vi "Newport PM-USB Dual CH 2936R.vi"(0 "Device State Control":T2, 1 "2936R Ref In":refnum<k24>, 5 "USB Address":i32=1, 7 "Remote Msg On":bool, 9 "PowerMeter 2936R Settings":T1={"Wavelength nm"=266, "Range Select"=0, "Mode"=0, "Unit Select"=2, "Auto Select"=1, "Analog Filter"=0, "Digital Filter\n(int. 0 to 10000)"=0, "Filter"=0} {"Filter" items=["No filtering", "Analog filter", "Digital filter", "Analog and Digital filter"]; "Digital Filter\n(int. 0 to 10000)" min=0 max=10000; "Analog Filter" items=["None", "250 kHz", "12.5 kHz", "1 kHz", "5 kHz"]; "Auto Select" items=["Manual Range", "Auto Range"]; "Unit Select" items=["Amps", "Volts", "Watts", "Watts/cm2", "Joules", "Joules/cm2", "dBm"]; "Mode" items=["CW Cont.", "DC Single", "Integrate", "Peak-to-Peak Cont.", "Peak-to-Peak Single", "Pulse Continuous", "Pulse Single", "RMS"]; "Range Select" items=["Range 0", "Range 1", "Range 2", "Range 3", "Range 4", "Range 5", "Range 6", "Range 7"]; "Wavelength nm" min=0}, 11 "2936R error in":errorcluster, 12 "Msg Ctl Refnum":refnum<vi>) -> (3 "2936R Ref Out":refnum<k24>, 4 "CH1, W":dbl, 6 "Ch2, W":dbl, 8 "Open USB IDs":string, 10 "Msg":string="\n\r" caption="Status", 13 "Error":bool, 14 "2936R Open?":bool, 15 "2936R error out":errorcluster)   [LabVIEW 2017]
uses:
  C:/Program Files (x86)/Newport/Newport USB Driver/Bin/UsbDllWrap.dll
  Program Files (x86)/Newport/Newport USB Driver/Bin/UsbDllWrap.dll
  Device State Control.ctl
panel:
  in  "Enable Error Reporting":bool=TRUE
  # "Model 1931-C|1936-C = Single Channel\nModel 2936-R = Dual Channel"
  # "Dual channel 2936R settings and power reading command"
  # "Ref out after init"
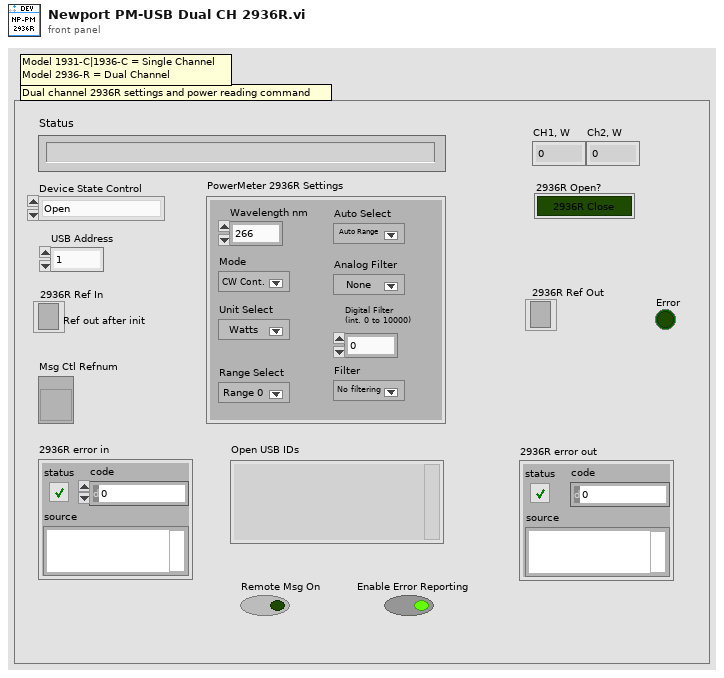
[diagram p1: front panel]
types:
  T1 = cluster{"Wavelength nm":i32, "Range Select":i32, "Mode":i32, "Unit Select":i32, "Auto Select":i32, "Analog Filter":i32, "Digital Filter\n(int. 0 to 10000)":i32, "Filter":i32}
  T2 = typedef "Device State Control.ctl" = enum16{"Open", "Close", "Clear", "Set", "Reset", "Read", "Write", "Call"}
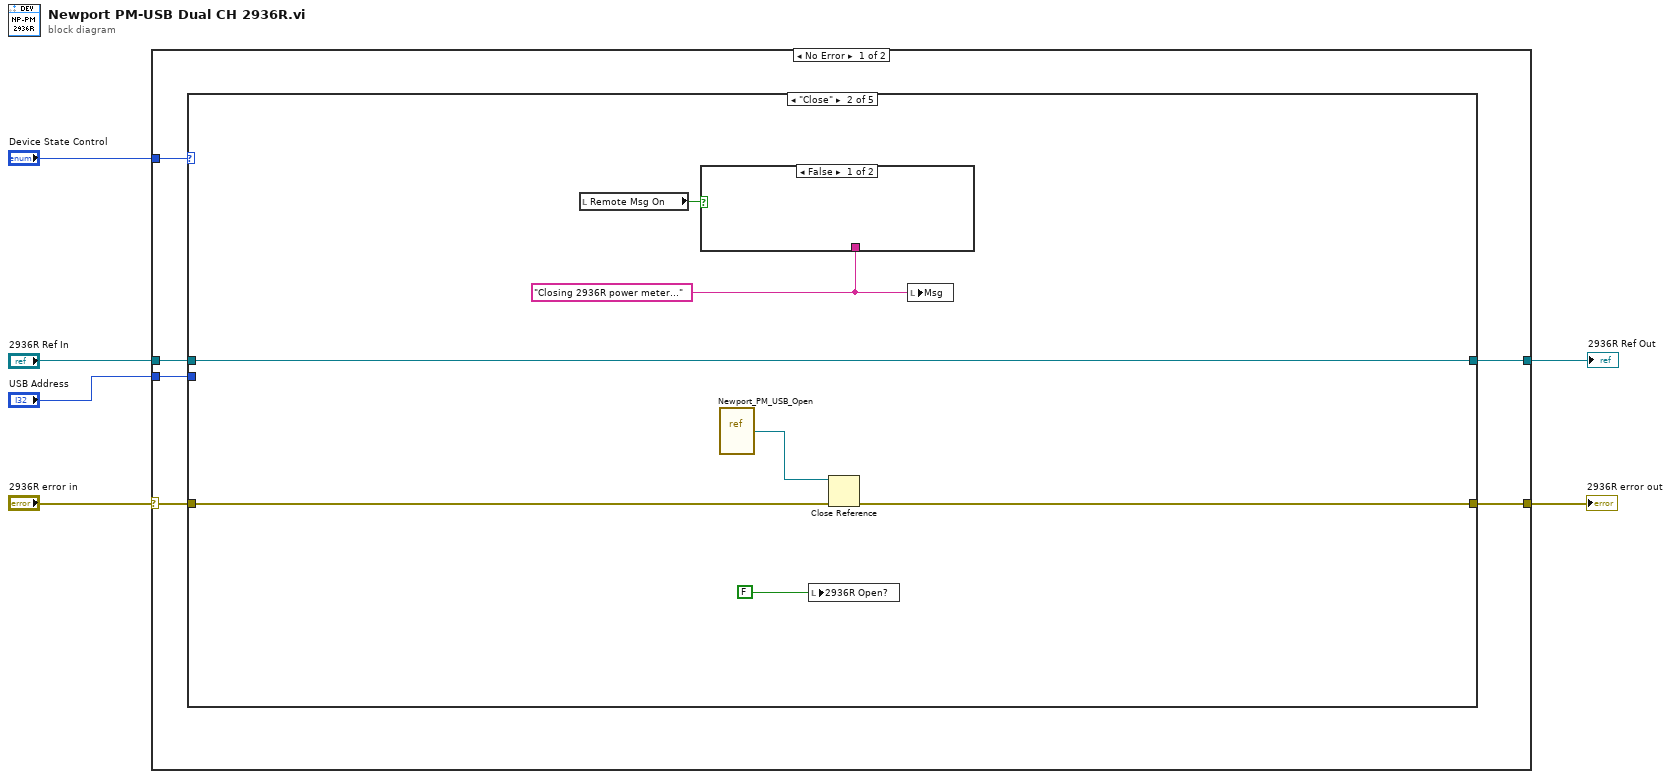
[diagram p0: block diagram]
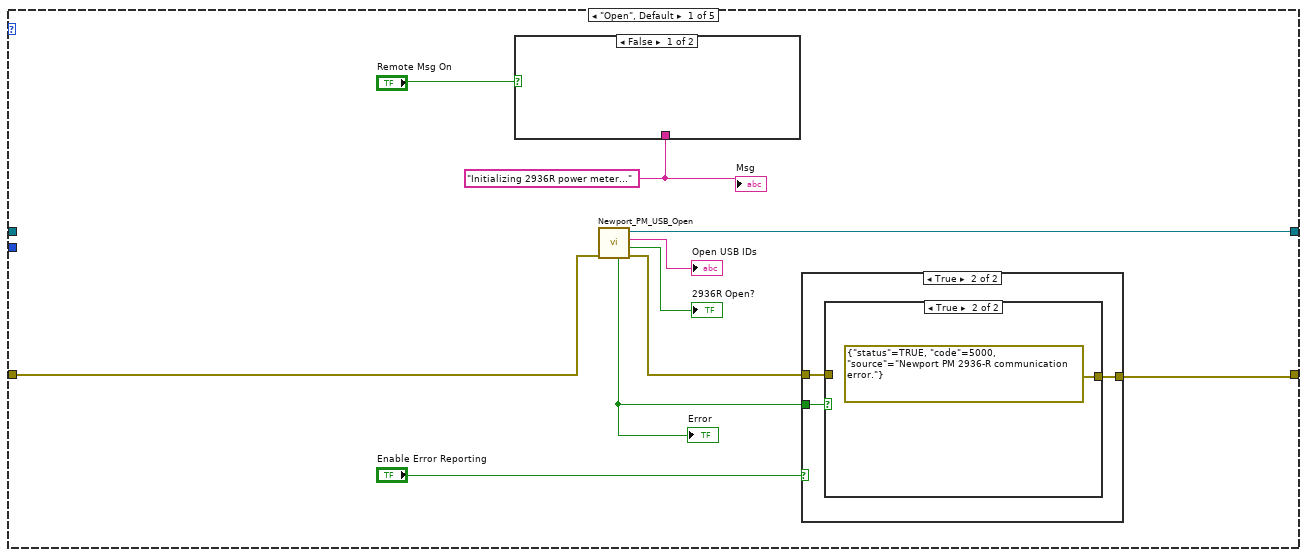
[diagram p2: hidden frame]
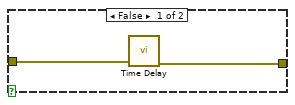
[diagram p4: hidden frame]
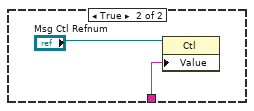
[diagram p5: hidden frame]
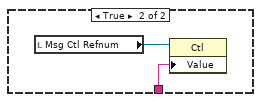
[diagram p6: hidden frame]
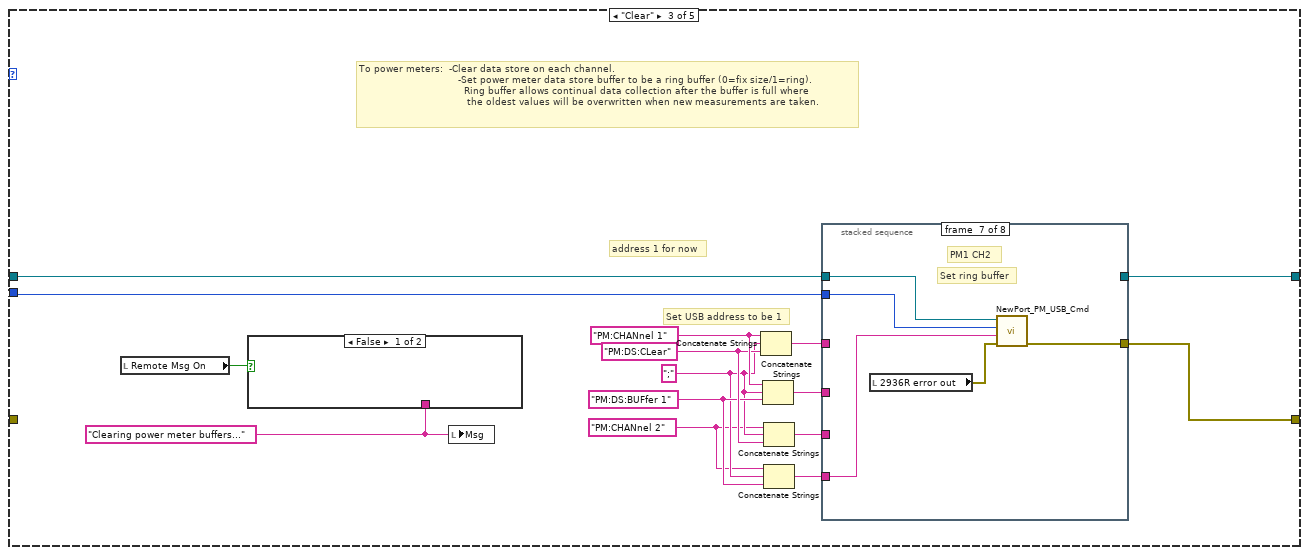
[diagram p7: hidden frame]
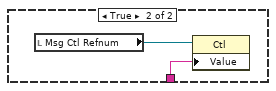
[diagram p8: hidden frame]
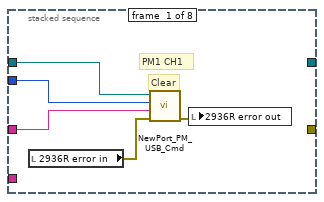
[diagram p9: hidden frame]
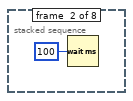
[diagram p10: hidden frame]
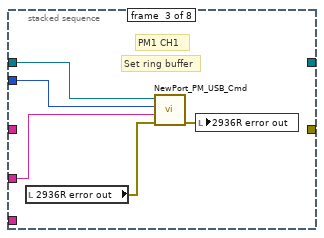
[diagram p11: hidden frame]
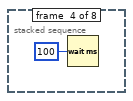
[diagram p12: hidden frame]
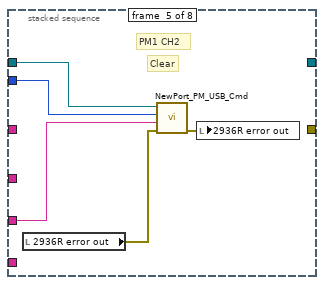
[diagram p13: hidden frame]
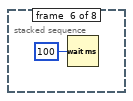
[diagram p14: hidden frame]
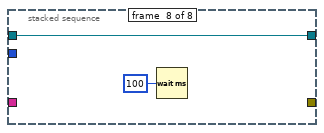
[diagram p15: hidden frame]
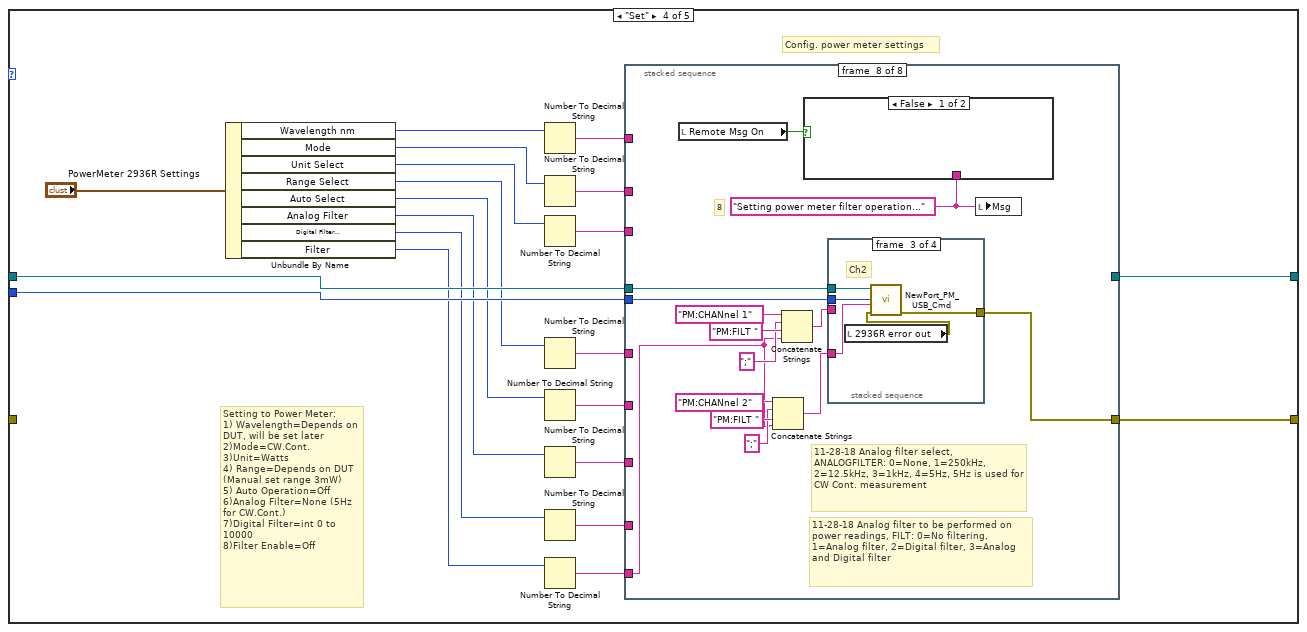
[diagram p16: hidden frame]
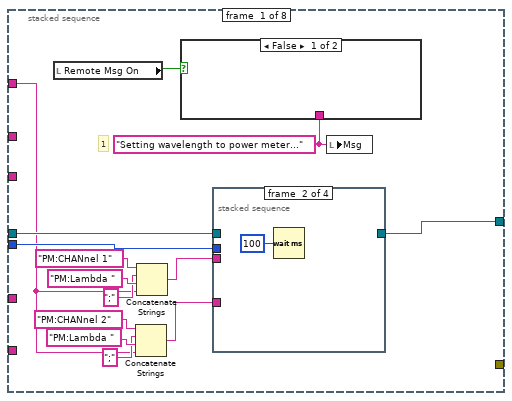
[diagram p17: hidden frame]
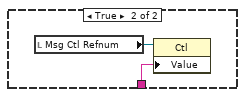
[diagram p18: hidden frame]
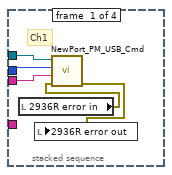
[diagram p19: hidden frame]
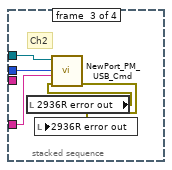
[diagram p20: hidden frame]
diagram:
  n1 = case shown="No Error" "2936R error in" {
    selector: "2936R error in" -> [w8 w349]
    tunnel: "Device State Control" -> [w12 _]
    tunnel: [w11 w350] -> w5
    tunnel: "2936R Ref In" -> [w10 w350]
    tunnel: "USB Address" -> [w9 _]
    tunnel: [w7 w349] -> w1
    frame No Error {
      n2 = case shown="\"Close\"" w12 {
        tunnel: w10 -> [_ w34 w45 w103 w332]
        tunnel: w9 -> [_ _ w46 w102 w336]
        tunnel: [w22 w34 w42 w101 w332] -> w11
        tunnel: w8 -> [w14 w33 _ _ _]
        tunnel: [w13 w32 w41 w83 w323] -> w7
        frame "Open", Default {
          w20 = "Initializing 2936R power meter..." ("Msg")
          n3 = case shown="False" "Remote Msg On" {
            tunnel: w20 -> [_ w31]
            frame False {
            }
            frame True {
              n4 = property class="Ctl"(reference="Msg Ctl Refnum", "Value"=w31) -> ()  [unwired: 1 in, 2 out]
            }
          }
          n5 = call "Newport_PM_USB_Open.vi"("Error In"=w14) -> ("error out"=w17:errorcluster, "OpenDevices"=→"2936R Open?":bool, "Output:"=→"Open USB IDs":string, "new reference"=w22:refnum<k24>, "Error"=w16:bool)  [unwired: 6 in]
          "Error" <- w16
          n6 = case shown="True" "Enable Error Reporting" {
            tunnel: w17 -> [w23 w26]
            tunnel: [w23 w25] -> w13
            tunnel: w16 -> [_ w24]
            frame False {
            }
            frame True {
              n7 = case shown="True" w24 {
                tunnel: w26 -> [w28 _]
                tunnel: [w27 errorcluster {"status"=TRUE, "code"=5000, "source"="Newport PM 2936-R communication error."} ("error constant")] -> w25
                frame False {
                  n8 = call "Time Delay"("error in (no error)"=w28) -> ("error out"=w27:errorcluster)  [unwired: 10 in]
                }
                frame True {
                }
              }
            }
          }
          "Msg" <- w20
        }
        frame "Close" {
          w37 = "Closing 2936R power meter..." ("Msg")
          n9 = local read "Remote Msg On"() -> (w35:bool)
          n10 = case shown="False" w35 {
            tunnel: w37 -> [_ w39]
            frame False {
            }
            frame True {
              n11 = local read "Msg Ctl Refnum"() -> (w40:refnum<vi>)
              n12 = property class="Ctl"(reference=w40, "Value"=w39) -> ()  [unwired: 1 in, 2 out]
            }
          }
          n13 = vi-ref "Newport_PM_USB_Open.vi"() -> (w36:refnum<vi>)
          n14 = local write "2936R Open?"(FALSE ("2936R Open?")) -> ()
          n15 = Close Reference(reference=w36, error in (no error)=w33) -> (error out=w32:errorcluster)
          n16 = local write "Msg"(w37) -> ()
        }
        frame "Clear" {
          w44 = "Clearing power meter buffers..." ("Msg")
          w51 = "PM:CHANnel 2" ("PM:CMD_QUERY In")
          w53 = "PM:DS:BUFfer 1" ("PM:CMD_QUERY In")
          w52 = ";" ("PM:CMD_QUERY In")
          w54 = "PM:DS:CLear" ("PM:CMD_QUERY In")
          w55 = "PM:CHANnel 1" ("PM:CMD_QUERY In")
          # "To power meters:  -Clear data store on each channel.\n                                 -Set power meter data store buffer to be a ring buffer (0=fix size/1=ring).  \n                                   Ring buffer allows continual data collection after the buffer is full where \n                                    the oldest values will be overwritten when new measurements are taken."
          # "address 1 for now"
          # "Set USB address to be 1"
          n17 = local read "Remote Msg On"() -> (w43:bool)
          n18 = case shown="False" w43 {
            tunnel: w44 -> [_ w56]
            frame False {
            }
            frame True {
              n19 = local read "Msg Ctl Refnum"() -> (w57:refnum<vi>)
              n20 = property class="Ctl"(reference=w57, "Value"=w56) -> ()  [unwired: 1 in, 2 out]
            }
          }
          n21 = local write "Msg"(w44) -> ()
          n22 = Concatenate Strings(w55, w52, w54) -> (w50:string)
          n23 = Concatenate Strings(w55, w52, w53) -> (w49:string)
          n24 = Concatenate Strings(w51, w52, w54) -> (w48:string)
          n25 = Concatenate Strings(w51, w52, w53) -> (w47:string)
          n26 = stacked-sequence {
            tunnel: w45 -> [w62 _ w68 _ w74 _ w78 w81]
            tunnel: w46 -> [w61 _ w67 _ w73 _ w79 _]
            tunnel: w50 -> [w60 _ _ _ _ _ _ _]
            tunnel: w49 -> [_ _ w66 _ _ _ _ _]
            tunnel: w48 -> [_ _ _ _ w72 _ _ _]
            tunnel: w47 -> [_ _ _ _ _ _ w80 _]
            tunnel: [_ _ _ _ _ _ _ w81] -> w42
            tunnel: [_ _ _ _ _ _ w76 _] -> w41
            frame #0 {
              # "Clear"
              # "PM1 CH1"
              n27 = local read "2936R error in"() -> (w58:errorcluster)
              n28 = call "NewPort_PM_USB_Cmd.vi"("error in"=w58, "PM:CMD_QUERY In"=w60, "USB Address"=w61, "reference"=w62) -> ("Error Out"=w59:errorcluster)  [unwired: 5 in, 2 out]
              n29 = local write "2936R error out"(w59) -> ()
            }
            frame #1 {
              n30 = Wait (ms)(milliseconds to wait=u32 100) -> ()  [unwired: 1 out]
            }
            frame #2 {
              # "Set ring buffer"
              # "PM1 CH1"
              n31 = local read "2936R error out"() -> (w64:errorcluster)
              n32 = call "NewPort_PM_USB_Cmd.vi"("error in"=w64, "PM:CMD_QUERY In"=w66, "USB Address"=w67, "reference"=w68) -> ("Error Out"=w65:errorcluster)  [unwired: 5 in, 2 out]
              n33 = local write "2936R error out"(w65) -> ()
            }
            frame #3 {
              n34 = Wait (ms)(milliseconds to wait=u32 100) -> ()  [unwired: 1 out]
            }
            frame #4 {
              # "Clear"
              # "PM1 CH2"
              n35 = local read "2936R error out"() -> (w70:errorcluster)
              n36 = call "NewPort_PM_USB_Cmd.vi"("error in"=w70, "PM:CMD_QUERY In"=w72, "USB Address"=w73, "reference"=w74) -> ("Error Out"=w71:errorcluster)  [unwired: 5 in, 2 out]
              n37 = local write "2936R error out"(w71) -> ()
            }
            frame #5 {
              n38 = Wait (ms)(milliseconds to wait=u32 100) -> ()  [unwired: 1 out]
            }
            frame #6 {
              # "Set ring buffer"
              # "PM1 CH2"
              n39 = local read "2936R error out"() -> (w77:errorcluster)
              n40 = call "NewPort_PM_USB_Cmd.vi"("error in"=w77, "PM:CMD_QUERY In"=w80, "USB Address"=w79, "reference"=w78) -> ("Error Out"=w76:errorcluster)  [unwired: 5 in, 2 out]
            }
            frame #7 {
              n41 = Wait (ms)(milliseconds to wait=u32 100) -> ()  [unwired: 1 out]
            }
          }
        }
        frame "Set" {
          # "Setting to Power Meter:\n1) Wavelength=Depends on DUT, will be set later\n2)Mode=CW.Cont.\n3)Unit=Watts\n4) Range=Depends on DUT (Manual set range 3mW)\n5) Auto Operation=Off\n6)Analog Filter=None (5Hz for CW.Cont.)\n7)Digital Filter=int 0 to 10000\n8)Filter Enable=Off"
          # "Config. power meter settings"
          n42 = Unbundle By Name("PowerMeter 2936R Settings") -> ("Wavelength nm"=w92:i32, "Mode"=w94:i32, "Unit Select"=w95:i32, "Range Select"=w96:i32, "Auto Select"=w97:i32, "Analog Filter"=w98:i32, "Digital Filter\n(int. 0 to 10000)"=w99:i32, "Filter"=w100:i32)
          n43 = Number To Decimal String(number=w92) -> (decimal integer string=w89:string)  [unwired: 1 in]
          n44 = Number To Decimal String(number=w94) -> (decimal integer string=w91:string)  [unwired: 1 in]
          n45 = Number To Decimal String(number=w95) -> (decimal integer string=w90:string)  [unwired: 1 in]
          n46 = Number To Decimal String(number=w96) -> (decimal integer string=w84:string)  [unwired: 1 in]
          n47 = Number To Decimal String(number=w97) -> (decimal integer string=w85:string)  [unwired: 1 in]
          n48 = Number To Decimal String(number=w98) -> (decimal integer string=w86:string)  [unwired: 1 in]
          n49 = Number To Decimal String(number=w99) -> (decimal integer string=w87:string)  [unwired: 1 in]
          n50 = Number To Decimal String(number=w100) -> (decimal integer string=w88:string)  [unwired: 1 in]
          n51 = stacked-sequence {
            tunnel: w102 -> [w111 w136 w163 w193 w217 w246 w273 w305]
            tunnel: w103 -> [w110 w137 w164 w192 w218 w247 w274 w306]
            tunnel: w84 -> [_ _ _ w189 _ _ _ _]
            tunnel: w85 -> [_ _ _ _ w216 _ _ _]
            tunnel: w86 -> [_ _ _ _ _ w243 _ _]
            tunnel: w87 -> [_ _ _ _ _ _ w272 _]
            tunnel: w88 -> [_ _ _ _ _ _ _ w298]
            tunnel: w89 -> [w107 _ _ _ _ _ _ _]
            tunnel: w90 -> [_ _ w162 _ _ _ _ _]
            tunnel: w91 -> [_ w135 _ _ _ _ _ _]
            tunnel: [w104 _ _ _ _ _ _ _] -> w101
            tunnel: [_ _ _ _ _ _ _ w295] -> w83
            frame #0 {
              w106 = "Setting wavelength to power meter..." ("Msg")
              # "1"
              n52 = local read "Remote Msg On"() -> (w105:bool)
              n53 = Concatenate Strings("PM:CHANnel 2" ("PM:CMD_QUERY In"), ";" ("PM:CMD_QUERY In"), "PM:Lambda " ("PM:CMD_QUERY In"), w107) -> (w117:string)
              n54 = Concatenate Strings("PM:CHANnel 1" ("PM:CMD_QUERY In"), ";" ("PM:CMD_QUERY In"), "PM:Lambda " ("PM:CMD_QUERY In"), w107) -> (w116:string)
              n55 = case shown="False" w105 {
                tunnel: w106 -> [_ w118]
                frame False {
                }
                frame True {
                  n56 = local read "Msg Ctl Refnum"() -> (w119:refnum<vi>)
                  n57 = property class="Ctl"(reference=w119, "Value"=w118) -> ()  [unwired: 1 in, 2 out]
                }
              }
              n58 = stacked-sequence {
                tunnel: w110 -> [w124 _ w130 w131]
                tunnel: w111 -> [w123 _ w129 _]
                tunnel: w116 -> [w122 _ _ _]
                tunnel: w117 -> [_ _ w128 _]
                tunnel: [_ _ _ w131] -> w104
                frame #0 {
                  # "Ch1"
                  n59 = local read "2936R error in"() -> (w121:errorcluster)
                  n60 = call "NewPort_PM_USB_Cmd.vi"("error in"=w121, "PM:CMD_QUERY In"=w122, "USB Address"=w123, "reference"=w124) -> ("Error Out"=w120:errorcluster)  [unwired: 5 in, 2 out]
                  n61 = local write "2936R error out"(w120) -> ()
                }
                frame #1 {
                  n62 = Wait (ms)(milliseconds to wait=u32 100) -> ()  [unwired: 1 out]
                }
                frame #2 {
                  # "Ch2"
                  n63 = local read "2936R error out"() -> (w127:errorcluster)
                  n64 = call "NewPort_PM_USB_Cmd.vi"("error in"=w127, "PM:CMD_QUERY In"=w128, "USB Address"=w129, "reference"=w130) -> ("Error Out"=w126:errorcluster)  [unwired: 5 in, 2 out]
                  n65 = local write "2936R error out"(w126) -> ()
                }
                frame #3 {
                  n66 = Wait (ms)(milliseconds to wait=u32 100) -> ()  [unwired: 1 out]
                }
              }
              n67 = local write "Msg"(w106) -> ()
            }
            frame #1 {
              w134 = "Setting power meter mode..." ("Msg")
              # "2"
              # "11-28-18 Mode select, MODE: \n0 DC Continuous =CW Cont.\n1 DC Single\n2 Integrate\n3 Peak-to-peak Continuous\n4 Peak-to-peak Single\n5 Pulse Continuous\n6 Pulse Single\n7 RMS"
              n68 = local read "Remote Msg On"() -> (w133:bool)
              n69 = case shown="False" w133 {
                tunnel: w134 -> [_ w146]
                frame False {
                }
                frame True {
                  n70 = local read "Msg Ctl Refnum"() -> (w147:refnum<vi>)
                  n71 = property class="Ctl"(reference=w147, "Value"=w146) -> ()  [unwired: 1 in, 2 out]
                }
              }
              n72 = Concatenate Strings("PM:CHANnel 2" ("PM:CMD_QUERY In"), ";" ("PM:CMD_QUERY In"), "PM:MODE 0" ("PM:CMD_QUERY In"), w135) -> (w145:string)
              n73 = Concatenate Strings("PM:CHANnel 1" ("PM:CMD_QUERY In"), ";" ("PM:CMD_QUERY In"), "PM:MODE 0" ("PM:CMD_QUERY In"), w135) -> (w144:string)
              n74 = stacked-sequence {
                tunnel: w137 -> [w152 _ w158 _]
                tunnel: w136 -> [w151 _ w157 _]
                tunnel: w144 -> [w150 _ _ _]
                tunnel: w145 -> [_ _ w156 _]
                frame #0 {
                  # "Ch1"
                  n75 = local read "2936R error out"() -> (w149:errorcluster)
                  n76 = call "NewPort_PM_USB_Cmd.vi"("error in"=w149, "PM:CMD_QUERY In"=w150, "USB Address"=w151, "reference"=w152) -> ("Error Out"=w148:errorcluster)  [unwired: 5 in, 2 out]
                  n77 = local write "2936R error out"(w148) -> ()
                }
                frame #1 {
                  n78 = Wait (ms)(milliseconds to wait=u32 100) -> ()  [unwired: 1 out]
                }
                frame #2 {
                  # "Ch2"
                  n79 = local read "2936R error out"() -> (w155:errorcluster)
                  n80 = call "NewPort_PM_USB_Cmd.vi"("error in"=w155, "PM:CMD_QUERY In"=w156, "USB Address"=w157, "reference"=w158) -> ("Error Out"=w154:errorcluster)  [unwired: 5 in, 2 out]
                  n81 = local write "2936R error out"(w154) -> ()
                }
                frame #3 {
                  n82 = Wait (ms)(milliseconds to wait=u32 100) -> ()  [unwired: 1 out]
                }
              }
              n83 = local write "Msg"(w134) -> ()
            }
            frame #2 {
              w161 = "Setting power meter unit..." ("Msg")
              # "3"
              # "11-28-18 Units select, UNITS: \n0 Amps\n1 Volts\n2 Watts\n3 Watts/cm2\n4 Joules\n5 Joules/cm2\n6 dBm\n7-10 Reserved\n11 Sun"
              n84 = local read "Remote Msg On"() -> (w160:bool)
              n85 = case shown="False" w160 {
                tunnel: w161 -> [_ w173]
                frame False {
                }
                frame True {
                  n86 = local read "Msg Ctl Refnum"() -> (w174:refnum<vi>)
                  n87 = property class="Ctl"(reference=w174, "Value"=w173) -> ()  [unwired: 1 in, 2 out]
                }
              }
              n88 = Concatenate Strings("PM:CHANnel 2" ("PM:CMD_QUERY In"), ";" ("PM:CMD_QUERY In"), "PM:UNITS " ("PM:CMD_QUERY In"), w162) -> (w172:string)
              n89 = Concatenate Strings("PM:CHANnel 1" ("PM:CMD_QUERY In"), ";" ("PM:CMD_QUERY In"), "PM:UNITS " ("PM:CMD_QUERY In"), w162) -> (w171:string)
              n90 = stacked-sequence {
                tunnel: w164 -> [w179 _ w185 _]
                tunnel: w163 -> [w178 _ w184 _]
                tunnel: w171 -> [w177 _ _ _]
                tunnel: w172 -> [_ _ w183 _]
                frame #0 {
                  # "Ch1"
                  n91 = local read "2936R error out"() -> (w176:errorcluster)
                  n92 = call "NewPort_PM_USB_Cmd.vi"("error in"=w176, "PM:CMD_QUERY In"=w177, "USB Address"=w178, "reference"=w179) -> ("Error Out"=w175:errorcluster)  [unwired: 5 in, 2 out]
                  n93 = local write "2936R error out"(w175) -> ()
                }
                frame #1 {
                  n94 = Wait (ms)(milliseconds to wait=u32 100) -> ()  [unwired: 1 out]
                }
                frame #2 {
                  # "Ch2"
                  n95 = local read "2936R error out"() -> (w182:errorcluster)
                  n96 = call "NewPort_PM_USB_Cmd.vi"("error in"=w182, "PM:CMD_QUERY In"=w183, "USB Address"=w184, "reference"=w185) -> ("Error Out"=w181:errorcluster)  [unwired: 5 in, 2 out]
                  n97 = local write "2936R error out"(w181) -> ()
                }
                frame #3 {
                  n98 = Wait (ms)(milliseconds to wait=u32 100) -> ()  [unwired: 1 out]
                }
              }
              n99 = local write "Msg"(w161) -> ()
            }
            frame #3 {
              w188 = "Setting power meter power range..." ("Msg")
              # "11-28-18 Power range select, RANge: \nThe PM:RANge command selects the gain stage when\nmaking readings from the detector head. The range of this\nvalue depends on the detector being used.\n\nint Values range from 0 to 7.  Detector in use is 918D-IS-1 2179 for NIR and FIR, the 8 ranges are, 0=387.3nW, 1=3.873uW,2=38.73uW, 3=387.3uW, 4=3.873mW, 5=38.73mW, 6=387.3mW, 7=3.873W. (10X greater from previous stage to the next, starting with stage 0)  Select 4."
              # "4"
              n100 = local read "Remote Msg On"() -> (w187:bool)
              n101 = Concatenate Strings("PM:CHANnel 2" ("PM:CMD_QUERY In"), ";" ("PM:CMD_QUERY In"), "PM:RAN " ("PM:CMD_QUERY In"), w189) -> (w199:string)
              n102 = Concatenate Strings("PM:CHANnel 1" ("PM:CMD_QUERY In"), ";" ("PM:CMD_QUERY In"), "PM:RAN " ("PM:CMD_QUERY In"), w189) -> (w198:string)
              n103 = case shown="False" w187 {
                tunnel: w188 -> [_ w200]
                frame False {
                }
                frame True {
                  n104 = local read "Msg Ctl Refnum"() -> (w201:refnum<vi>)
                  n105 = property class="Ctl"(reference=w201, "Value"=w200) -> ()  [unwired: 1 in, 2 out]
                }
              }
              n106 = stacked-sequence {
                tunnel: w192 -> [w206 _ w212 _]
                tunnel: w193 -> [w205 _ w211 _]
                tunnel: w198 -> [w204 _ _ _]
                tunnel: w199 -> [_ _ w210 _]
                frame #0 {
                  # "Ch1"
                  n107 = local read "2936R error out"() -> (w203:errorcluster)
                  n108 = call "NewPort_PM_USB_Cmd.vi"("error in"=w203, "PM:CMD_QUERY In"=w204, "USB Address"=w205, "reference"=w206) -> ("Error Out"=w202:errorcluster)  [unwired: 5 in, 2 out]
                  n109 = local write "2936R error out"(w202) -> ()
                }
                frame #1 {
                  n110 = Wait (ms)(milliseconds to wait=u32 100) -> ()  [unwired: 1 out]
                }
                frame #2 {
                  # "Ch2"
                  n111 = local read "2936R error out"() -> (w209:errorcluster)
                  n112 = call "NewPort_PM_USB_Cmd.vi"("error in"=w209, "PM:CMD_QUERY In"=w210, "USB Address"=w211, "reference"=w212) -> ("Error Out"=w208:errorcluster)  [unwired: 5 in, 2 out]
                  n113 = local write "2936R error out"(w208) -> ()
                }
                frame #3 {
                  n114 = Wait (ms)(milliseconds to wait=u32 100) -> ()  [unwired: 1 out]
                }
              }
              n115 = local write "Msg"(w188) -> ()
            }
            frame #4 {
              w215 = "Setting power meter auto operation..." ("Msg")
              # "5"
              # "11-28-18 Auto range select, AUTO: \n0=Manual power meter ranging\n1=Automatic power meter ranging"
              n116 = local read "Remote Msg On"() -> (w214:bool)
              n117 = Concatenate Strings("PM:CHANnel 2" ("PM:CMD_QUERY In"), ";" ("PM:CMD_QUERY In"), "PM:AUTO " ("PM:CMD_QUERY In"), w216) -> (w226:string)
              n118 = Concatenate Strings("PM:CHANnel 1" ("PM:CMD_QUERY In"), ";" ("PM:CMD_QUERY In"), "PM:AUTO " ("PM:CMD_QUERY In"), w216) -> (w225:string)
              n119 = case shown="False" w214 {
                tunnel: w215 -> [_ w227]
                frame False {
                }
                frame True {
                  n120 = local read "Msg Ctl Refnum"() -> (w228:refnum<vi>)
                  n121 = property class="Ctl"(reference=w228, "Value"=w227) -> ()  [unwired: 1 in, 2 out]
                }
              }
              n122 = stacked-sequence {
                tunnel: w218 -> [w233 _ w239 _]
                tunnel: w217 -> [w232 _ w238 _]
                tunnel: w225 -> [w231 _ _ _]
                tunnel: w226 -> [_ _ w237 _]
                frame #0 {
                  # "Ch1"
                  n123 = local read "2936R error out"() -> (w230:errorcluster)
                  n124 = call "NewPort_PM_USB_Cmd.vi"("error in"=w230, "PM:CMD_QUERY In"=w231, "USB Address"=w232, "reference"=w233) -> ("Error Out"=w229:errorcluster)  [unwired: 5 in, 2 out]
                  n125 = local write "2936R error out"(w229) -> ()
                }
                frame #1 {
                  n126 = Wait (ms)(milliseconds to wait=u32 100) -> ()  [unwired: 1 out]
                }
                frame #2 {
                  # "Ch2"
                  n127 = local read "2936R error out"() -> (w236:errorcluster)
                  n128 = call "NewPort_PM_USB_Cmd.vi"("error in"=w236, "PM:CMD_QUERY In"=w237, "USB Address"=w238, "reference"=w239) -> ("Error Out"=w235:errorcluster)  [unwired: 5 in, 2 out]
                  n129 = local write "2936R error out"(w235) -> ()
                }
                frame #3 {
                  n130 = Wait (ms)(milliseconds to wait=u32 100) -> ()  [unwired: 1 out]
                }
              }
              n131 = local write "Msg"(w215) -> ()
            }
            frame #5 {
              w242 = "Setting power meter analog filter..." ("Msg")
              # "6"
              # "Analog Filter frequency"
              # "11-28-18 Analog filter to be performed on power readings, FILT: 0=No filtering, 1=Analog filter, 2=Digital filter, 3=Analog and Digital filter"
              # "11-28-18 Analog filter select, ANALOGFILTER: 0=None, 1=250kHz, 2=12.5kHz, 3=1kHz, 4=5Hz, 5Hz is used for CW Cont. measurement"
              n132 = local read "Remote Msg On"() -> (w241:bool)
              n133 = Concatenate Strings("PM:CHANnel 1" ("PM:CMD_QUERY In"), ";" ("PM:CMD_QUERY In"), "PM:ANALOGFILTER " ("PM:CMD_QUERY In"), w243) -> (w251:string)
              n134 = Concatenate Strings("PM:CHANnel 2" ("PM:CMD_QUERY In"), ";" ("PM:CMD_QUERY In"), "PM:ANALOGFILTER " ("PM:CMD_QUERY In"), w243) -> (w248:string)
              n135 = stacked-sequence {
                tunnel: w247 -> [w260 _ w266 _]
                tunnel: w246 -> [w259 _ w265 _]
                tunnel: w251 -> [w258 _ _ _]
                tunnel: w248 -> [_ _ w264 _]
                frame #0 {
                  # "Ch1"
                  n136 = local read "2936R error out"() -> (w257:errorcluster)
                  n137 = call "NewPort_PM_USB_Cmd.vi"("error in"=w257, "PM:CMD_QUERY In"=w258, "USB Address"=w259, "reference"=w260) -> ("Error Out"=w256:errorcluster)  [unwired: 5 in, 2 out]
                  n138 = local write "2936R error out"(w256) -> ()
                }
                frame #1 {
                  n139 = Wait (ms)(milliseconds to wait=u32 100) -> ()  [unwired: 1 out]
                }
                frame #2 {
                  # "Ch2"
                  n140 = local read "2936R error out"() -> (w263:errorcluster)
                  n141 = call "NewPort_PM_USB_Cmd.vi"("error in"=w263, "PM:CMD_QUERY In"=w264, "USB Address"=w265, "reference"=w266) -> ("Error Out"=w262:errorcluster)  [unwired: 5 in, 2 out]
                  n142 = local write "2936R error out"(w262) -> ()
                }
                frame #3 {
                  n143 = Wait (ms)(milliseconds to wait=u32 100) -> ()  [unwired: 1 out]
                }
              }
              n144 = case shown="False" w241 {
                tunnel: w242 -> [_ w254]
                frame False {
                }
                frame True {
                  n145 = local read "Msg Ctl Refnum"() -> (w255:refnum<vi>)
                  n146 = property class="Ctl"(reference=w255, "Value"=w254) -> ()  [unwired: 1 in, 2 out]
                }
              }
              n147 = local write "Msg"(w242) -> ()
            }
            frame #6 {
              w269 = "Setting power meter digital filter..." ("Msg")
              # "7"
              # "11-28-18 Digital filter select, DIGITALFILTER: int value digital filter size between 0 and 10000 measurement"
              n148 = local read "Remote Msg On"() -> (w268:bool)
              n149 = case shown="False" w268 {
                tunnel: w269 -> [_ w281]
                frame False {
                }
                frame True {
                  n150 = local read "Msg Ctl Refnum"() -> (w282:refnum<vi>)
                  n151 = property class="Ctl"(reference=w282, "Value"=w281) -> ()  [unwired: 1 in, 2 out]
                }
              }
              n152 = Concatenate Strings("PM:CHANnel 2" ("PM:CMD_QUERY In"), ";" ("PM:CMD_QUERY In"), "PM:DIGITALFILTER " ("PM:CMD_QUERY In"), w272) -> (w280:string)
              n153 = Concatenate Strings("PM:CHANnel 1" ("PM:CMD_QUERY In"), ";" ("PM:CMD_QUERY In"), "PM:DIGITALFILTER " ("PM:CMD_QUERY In"), w272) -> (w279:string)
              n154 = stacked-sequence {
                tunnel: w274 -> [w287 _ w293 _]
                tunnel: w273 -> [w286 _ w292 _]
                tunnel: w279 -> [w285 _ _ _]
                tunnel: w280 -> [_ _ w291 _]
                frame #0 {
                  # "Ch1"
                  n155 = local read "2936R error out"() -> (w284:errorcluster)
                  n156 = call "NewPort_PM_USB_Cmd.vi"("error in"=w284, "PM:CMD_QUERY In"=w285, "USB Address"=w286, "reference"=w287) -> ("Error Out"=w283:errorcluster)  [unwired: 5 in, 2 out]
                  n157 = local write "2936R error out"(w283) -> ()
                }
                frame #1 {
                  n158 = Wait (ms)(milliseconds to wait=u32 100) -> ()  [unwired: 1 out]
                }
                frame #2 {
                  # "Ch2"
                  n159 = local read "2936R error out"() -> (w290:errorcluster)
                  n160 = call "NewPort_PM_USB_Cmd.vi"("error in"=w290, "PM:CMD_QUERY In"=w291, "USB Address"=w292, "reference"=w293) -> ("Error Out"=w289:errorcluster)  [unwired: 5 in, 2 out]
                  n161 = local write "2936R error out"(w289) -> ()
                }
                frame #3 {
                  n162 = Wait (ms)(milliseconds to wait=u32 100) -> ()  [unwired: 1 out]
                }
              }
              n163 = local write "Msg"(w269) -> ()
            }
            frame #7 {
              w297 = "Setting power meter filter operation..." ("Msg")
              # "8"
              # "11-28-18 Analog filter to be performed on power readings, FILT: 0=No filtering, 1=Analog filter, 2=Digital filter, 3=Analog and Digital filter"
              # "11-28-18 Analog filter select, ANALOGFILTER: 0=None, 1=250kHz, 2=12.5kHz, 3=1kHz, 4=5Hz, 5Hz is used for CW Cont. measurement"
              n164 = local read "Remote Msg On"() -> (w296:bool)
              n165 = Concatenate Strings("PM:CHANnel 2" ("PM:CMD_QUERY In"), ";" ("PM:CMD_QUERY In"), "PM:FILT " ("PM:CMD_QUERY In"), w298) -> (w307:string)
              n166 = Concatenate Strings("PM:CHANnel 1" ("PM:CMD_QUERY In"), ";" ("PM:CMD_QUERY In"), "PM:FILT " ("PM:CMD_QUERY In"), w298) -> (w308:string)
              n167 = case shown="False" w296 {
                tunnel: w297 -> [_ w309]
                frame False {
                }
                frame True {
                  n168 = local read "Msg Ctl Refnum"() -> (w310:refnum<vi>)
                  n169 = property class="Ctl"(reference=w310, "Value"=w309) -> ()  [unwired: 1 in, 2 out]
                }
              }
              n170 = stacked-sequence {
                tunnel: w306 -> [w315 _ w321 _]
                tunnel: w305 -> [w314 _ w320 _]
                tunnel: w308 -> [w313 _ _ _]
                tunnel: w307 -> [_ _ w319 _]
                tunnel: [_ _ w317 _] -> w295
                frame #0 {
                  # "Ch1"
                  n171 = local read "2936R error out"() -> (w312:errorcluster)
                  n172 = call "NewPort_PM_USB_Cmd.vi"("error in"=w312, "PM:CMD_QUERY In"=w313, "USB Address"=w314, "reference"=w315) -> ("Error Out"=w311:errorcluster)  [unwired: 5 in, 2 out]
                  n173 = local write "2936R error out"(w311) -> ()
                }
                frame #1 {
                  n174 = Wait (ms)(milliseconds to wait=u32 100) -> ()  [unwired: 1 out]
                }
                frame #2 {
                  # "Ch2"
                  n175 = local read "2936R error out"() -> (w318:errorcluster)
                  n176 = call "NewPort_PM_USB_Cmd.vi"("error in"=w318, "PM:CMD_QUERY In"=w319, "USB Address"=w320, "reference"=w321) -> ("Error Out"=w317:errorcluster)  [unwired: 5 in, 2 out]
                }
                frame #3 {
                  n177 = Wait (ms)(milliseconds to wait=u32 100) -> ()  [unwired: 1 out]
                }
              }
              n178 = local write "Msg"(w297) -> ()
            }
          }
        }
        frame "Read" {
          w334 = "Getting power readings..." ("Msg")
          # "Ch2"
          # "Ch1"
          n179 = local read "2936R error in"() -> (w335:errorcluster)
          n180 = call "NewPort_PM_USB_Read-Set.vi"("reference"=w332, "USB Address"=w336, "Read Power(F)\nSet Lambda(T)"=FALSE ("Read Power(T)\nSet Lambda(F)"), "error in"=w335, "Read Power\nSingle CH(F)\nDual CHs(T)"=TRUE ("Set Lambda\nSingle CH(F)\nDual CHs(T)")) -> ("Query-String Format\nfrom Read Buffer"=w338:string, "error out"=w323:errorcluster)  [unwired: 9 in]
          n181 = Match Pattern(string=w338, regular expression=",") -> (before substring=w339:string, after substring=w340:string)  [unwired: 1 in, 2 out]
          n182 = local read "Remote Msg On"() -> (w333:bool)
          n183 = Fract/Exp String To Number(string=w340) -> (number=w324:dbl)  [unwired: 3 in, 1 out]
          n184 = case shown="False" w333 {
            tunnel: w334 -> [_ w347]
            frame False {
            }
            frame True {
              n185 = local read "Msg Ctl Refnum"() -> (w348:refnum<vi>)
              n186 = property class="Ctl"(reference=w348, "Value"=w347) -> ()  [unwired: 1 in, 2 out]
            }
          }
          n187 = Fract/Exp String To Number(string=w339) -> (number=w329:dbl)  [unwired: 3 in, 1 out]
          n188 = Greater?(x=w329, y=100.0) -> (0:w331:bool)
          n189 = Greater?(x=w324, y=100.0) -> (0:w326:bool)
          n190 = local write "Msg"(w334) -> ()
          n191 = case shown="False" w331 {
            tunnel: w329 -> [w345 _]
            tunnel: [w345 0.0] -> w328
            frame False {
            }
            frame True {
            }
          }
          "CH1, W" <- w328
          n192 = case shown="True" w326 {
            tunnel: w324 -> [w343 _]
            tunnel: [w343 0.0] -> w325
            frame False {
            }
            frame True {
            }
          }
          "Ch2, W" <- w325
        }
      }
    }
    frame Error {
    }
  }
  "2936R Ref Out" <- w5
  "2936R error out" <- w1
